vi "Add row to database.vi"(8 "error in (no error)":errorcluster, 11 "Panel Form Controller in":refnum<class "Panel Form Controller.lvclass">) -> (0 "error out":errorcluster, 3 "Panel Form Controller out":refnum<class "Panel Form Controller.lvclass">)   [LabVIEW 2020, in "Panel Form Controller.lvlib" / "Panel Form Controller.lvclass"]
uses:
  Panel Form Controller.lvclass
  C:/Program Files (x86)/National Instruments/LabVIEW 2020/vi.lib/ActorFramework/Actor/Actor.lvclass
  Forms Server/Update Fields Logic/Field FK PK Info.ctl
  Panel Form Controller.lvclass/Panel Form Controller.ctl
  <vilib>/ActorFramework/Actor/Actor.lvclass/Actor.ctl
  Forms Model/Form Model Interfaces/Form Model Messages Messages/Request FK Update Msg/Request FK Update Msg.lvclass/Request FK Update Msg.ctl
  <vilib>/ActorFramework/Message Enqueuer/Message Enqueuer.lvclass/Message Enqueuer.ctl
  <vilib>/ActorFramework/Message Enqueuer/Enqueue.vi
  Database OOP/Table Libraries/Basic Form/Basic Form.lvclass
  C:/Users/User/Desktop/Raman Program/LV-Database-OOP/source/Database OOP/Table Libraries/Basic Table/Basic Table Class/Basic Table.lvclass
  Forms Model/Form Model Interfaces/Form Model Messages Messages/Request FK Update Msg/Request FK Update Msg.lvclass
  C:/Program Files (x86)/National Instruments/LabVIEW 2020/vi.lib/ActorFramework/Message/Message.lvclass
  <vilib>/ActorFramework/Message Priority Queue/Priority Enqueue.vi
  Database OOP/Table Libraries/Table Configuration Interface/Table Configuration Interface.lvclass
  Database OOP/Table Libraries/Basic Table/Basic Table Class/Basic Table.lvclass
  <vilib>/ActorFramework/Actor/Actor.lvclass
  Forms Server/Form Server Interfaces.lvlib
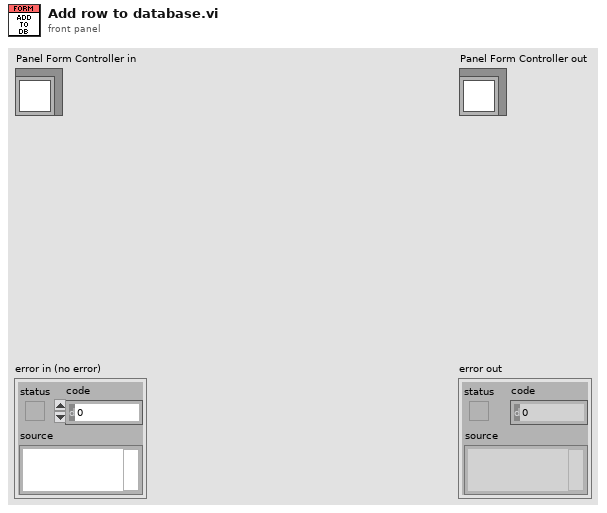
[diagram p1: front panel]
types:
  T1 = typedef "Form Server Interfaces.lvlib/Field FK PK Info.ctl" = cluster{"Field ID":string[], "FK Table":string[], "FK Column":string[], "PK Table":string[], "PK Column":string[]}
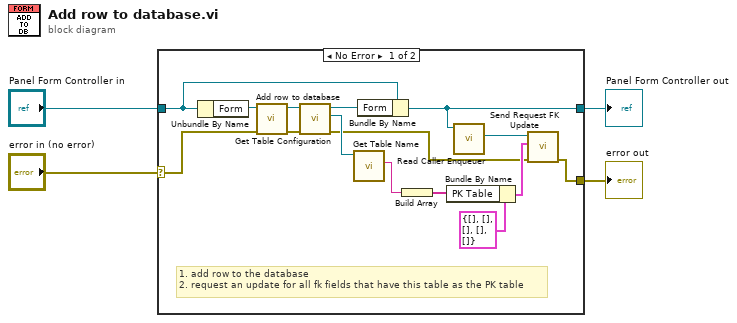
[diagram p0: block diagram]
diagram:
  n1 = case shown="No Error" "error in (no error)" {
    selector: "error in (no error)" -> [w18 w21]
    tunnel: [w5 w21] -> w3
    tunnel: [w17 w20] -> w1
    tunnel: "Panel Form Controller in" -> [w19 w20]
    frame No Error {
      # "1. add row to the database\n2. request an update for all fk fields that have this table as the PK table"
      n2 = Unbundle By Name(w19) -> ("Form"=w15:refnum<class "Basic Form.lvclass">)
      n3 = call "Add row to database.vi"("error in (no error)"=w18, "Basic Table in"=w15) -> ("error out"=w7:errorcluster, "Basic Table out"=w14:refnum<class "Basic Form.lvclass">)  [unwired: 8 in]
      n4 = call "Get Table Configuration.vi"("error in (no error)"=w7, "Basic Table in"=w14) -> ("error out"=w6:errorcluster, "Table Configuration"=w13:refnum<class "Table Configuration Interface.lvclass">, "Basic Table out"=w12:refnum<class "Basic Form.lvclass">)  [unwired: 7 in]
      n5 = call-dynamic "Get Table Name.vi"("Table Configuration Interface in"=w13) -> ("Table Name"=w10:string)  [unwired: 8 in, 2 out]
      n6 = Bundle By Name(cluster=w19, "Form"=w12) -> (w17:refnum<class "Panel Form Controller.lvclass">)
      n7 = Build Array(w10) -> (w9:string[])
      n8 = Bundle By Name(cluster=T1 {"Field ID"=[], "FK Table"=[], "FK Column"=[], "PK Table"=[], "PK Column"=[]} ("Filter FK/PK"), "PK Table"=w9) -> (w8:T1)
      n9 = call <vilib>:"Read Caller Enqueuer.vi"("Actor"=w17) -> ("Caller Enqueuer"=w16:refnum<class "Message Enqueuer.lvclass">)  [unwired: 10 in]
      n10 = call "Send Request FK Update.vi"("error in (no error)"=w6, "Filter FK/PK"=w8, "Message Enqueuer"=w16) -> ("error out"=w5:errorcluster)  [unwired: 7 in, 1 out]
    }
    frame Error {
    }
  }
  "error out" <- w3
  "Panel Form Controller out" <- w1
